vi "Set UIPosition.vi"(8 "error in":errorcluster, 9 "VI Ref":refnum<vi>, 11 "Sequence Context In":refnum<k7>) -> (0 "error out":errorcluster)   [LabVIEW 2021]
uses:
  Windows/System32/user32.dll
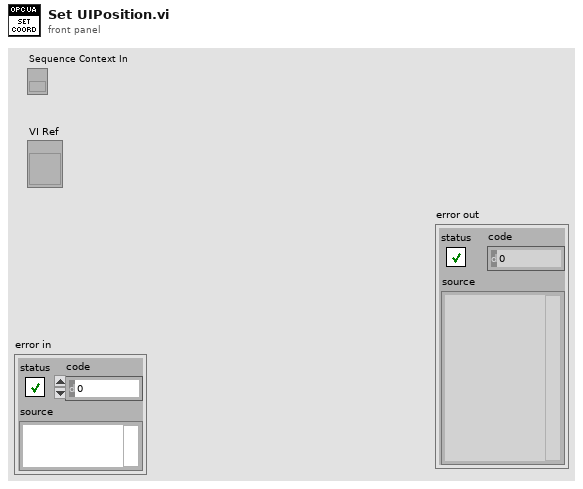
[diagram p1: front panel]
types:
  T1 = typedef "LVRectTypeDef.ctl" = cluster{"Left":i16, "Top":i16, "Right":i16, "Bottom":i16}
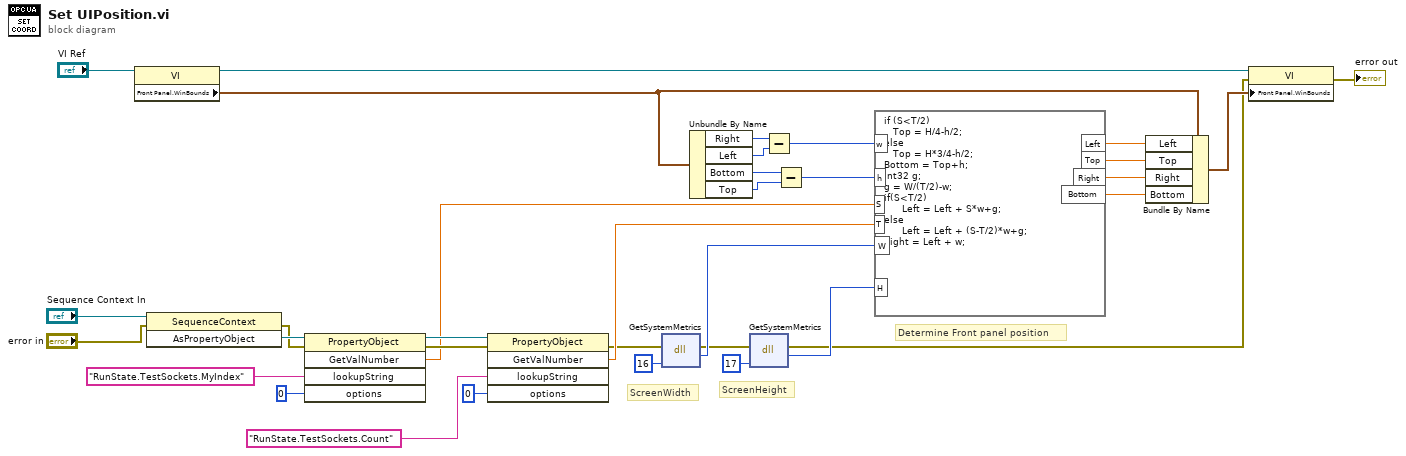
[diagram p0: block diagram]
diagram:
  # "Determine Front panel position"
  # "ScreenHeight"
  # "ScreenWidth"
  n1 = property class="VI"(reference="VI Ref") -> (reference out=w18:refnum<vi>, "Front Panel.WinBounds"=w17:T1)  [unwired: 1 in, 1 out]
  n2 = invoke class="SequenceContext" method="AsPropertyObject"(reference="Sequence Context In", error in="error in") -> (error out=w9:errorcluster, "AsPropertyObject"=w33:refnum<k7>)  [unwired: 1 in, 1 out]
  n3 = invoke class="PropertyObject" method="GetValNumber"(reference=w33, error in=w9, "lookupString"="RunState.TestSockets.MyIndex" ("Lookup String"), "options"=0) -> (reference out=w30:refnum<k7>, error out=w8:errorcluster, "GetValNumber"=w5:dbl)  [unwired: 1 in, 2 out]
  n4 = invoke class="PropertyObject" method="GetValNumber"(reference=w30, error in=w8, "lookupString"="RunState.TestSockets.Count" ("Lookup String"), "options"=0) -> (error out=w3:errorcluster, "GetValNumber"=w4:dbl)  [unwired: 1 in, 3 out]
  n5 = dll-call lib="C:/Windows/System32/user32.dll" fn="GetSystemMetrics"(error in=w3, "nIndex"=16) -> (error out=w7:errorcluster, "return type"=w24:i32)  [unwired: 3 in, 1 out]
  n6 = Unbundle By Name(w17) -> ("Right"=w16:i16, "Left"=w15:i16, "Bottom"=w13:i16, "Top"=w12:i16)
  n7 = dll-call lib="C:/Windows/System32/user32.dll" fn="GetSystemMetrics"(error in=w7, "nIndex"=17) -> (error out=w1:errorcluster, "return type"=w23:i32)  [unwired: 3 in, 1 out]
  n8 = Subtract(x=w16, y=w15) -> (x-y=w14:i16)
  n9 = Subtract(x=w13, y=w12) -> (x-y=w11:i16)
  n10 = formula code="if (S<T/2)\n   Top = H/4-h/2;\nelse\n   Top = H*3/4-h/2;\nBottom = Top+h;\nint32 g;\ng = W/(T/2)-w;\nif(S<T/2)\n      Left = Left + S*w+g;\nelse\n      Left = Left + (S-T/2)*w+g;\nRight = Left + w;"("S"=w5, "T"=w4, "W"=w24, "H"=w23, "w"=w14, "h"=w11) -> ("Left"=w22:dbl, "Top"=w21:dbl, "Right"=w20:dbl, "Bottom"=w19:dbl)
  n11 = Bundle By Name(cluster=w17, "Left"=w22, "Top"=w21, "Right"=w20, "Bottom"=w19) -> (w27:T1)
  n12 = property on="Property Node" class="VI"(reference=w18, error in=w1, "Front Panel.WinBounds"=w27) -> (error out=→"error out":errorcluster)  [unwired: 1 out]
